vi "Absolute Time Chart 2-LV12.vi"() -> ()   [LabVIEW 2012]
panel:
  out "Waveform Chart":waveform(dbl)(graph)
  in  "stop":bool
  in  "Samples Per Second":dbl=15.0
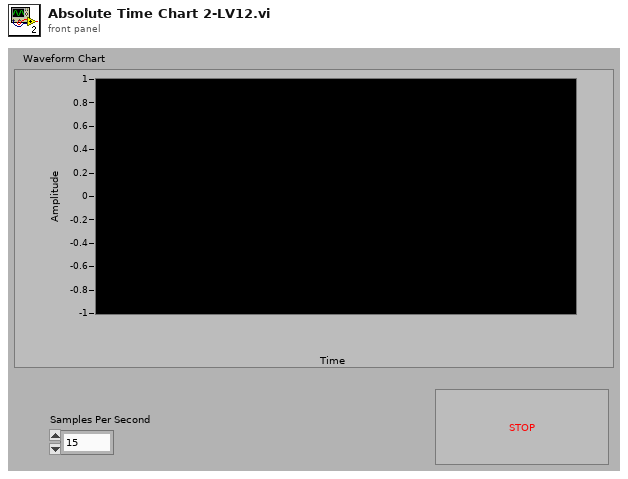
[diagram p1: front panel]
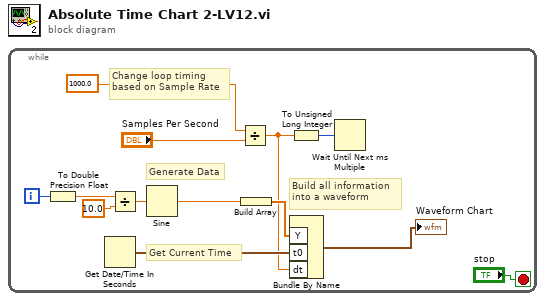
[diagram p0: block diagram]
diagram:
  n1 = while {
    i -> [w9]
    stop <- "stop" stop-if-true
    # "Build all information\ninto a waveform"
    # "Change loop timing\nbased on Sample Rate"
    # "Get Current Time"
    # "Generate Data"
    n2 = To Double Precision Float(number=w9) -> (double precision float=w8:dbl)
    n3 = Get Date/Time In Seconds() -> (seconds since 1Jan1904=w3:timestamp)
    n4 = Divide(x=w8, y=10.0) -> (x/y=w12:dbl)
    n5 = Sine(x=w12) -> (sin(x)=w5:dbl)
    n6 = Divide(x=1000.0, y="Samples Per Second") -> (x/y=w2:dbl)
    n7 = Build Array(w5) -> (w4:dbl[])
    n8 = Bundle By Name("Y"=w4, "t0"=w3, "dt"=w2) -> (→"Waveform Chart":waveform(dbl))  [unwired: 1 in]
    n9 = To Unsigned Long Integer(number=w2) -> (unsigned 32bit integer=w10:u32)
    n10 = Wait Until Next ms Multiple(millisecond multiple=w10) -> ()  [unwired: 1 out]
  }
